vi "Initialization.vi"(8 "error in (no error)":errorcluster, 11 "Messages Actor in":refnum<class "Messages Actor.lvclass">) -> (0 "error out":errorcluster, 3 "Messages Actor out":refnum<class "Messages Actor.lvclass">)   [LabVIEW 2020, in "Messages Actor.lvlib" / "Messages Actor.lvclass"]
uses:
  Messages Actor.lvclass
  Messages Actor.lvclass/Messages Actor.ctl
  Read Messages Sub Panel.vi
  Read VI Refnum.vi
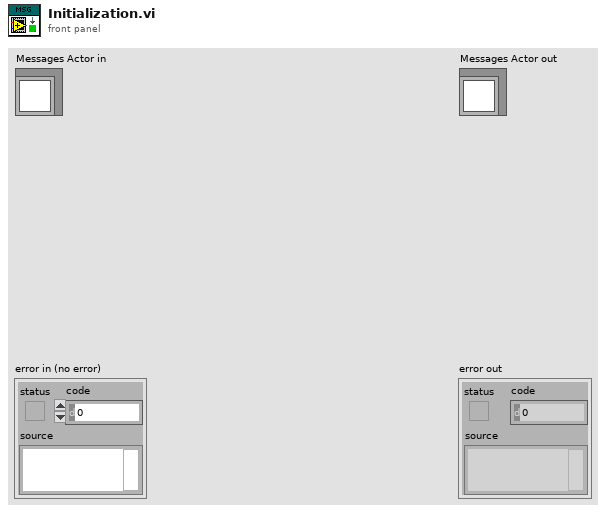
[diagram p1: front panel]
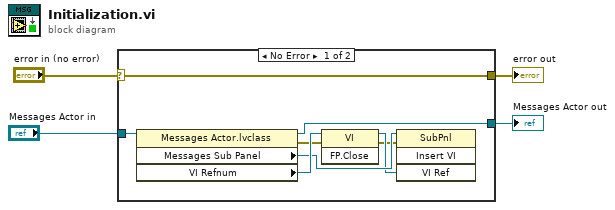
[diagram p0: block diagram]
diagram:
  n1 = case shown="No Error" "error in (no error)" {
    selector: "error in (no error)" -> [w11 w14]
    tunnel: [w11 w14] -> w3
    tunnel: [w10 w13] -> w1
    tunnel: "Messages Actor in" -> [w12 w13]
    frame No Error {
      n2 = property class="Messages Actor.lvclass"(reference=w12) -> (reference out=w10:refnum<class "Messages Actor.lvclass">, error out=w5:errorcluster, "Messages Sub Panel"=w8:refnum<vi>, "VI Refnum"=w9:refnum<vi>)  [unwired: 1 in]
      n3 = invoke class="VI" method="FP.Close"(reference=w9, error in=w5) -> (reference out=w7:refnum<vi>, error out=w6:errorcluster)  [unwired: 1 in, 1 out]
      n4 = invoke class="SubPnl" method="Insert VI"(reference=w8, error in=w6, "VI Ref"=w7) -> ()  [unwired: 1 in, 4 out]
    }
    frame Error {
    }
  }
  "error out" <- w3
  "Messages Actor out" <- w1
